vi "Project Save As.vi"(8 "error in (no error)":errorcluster, 9 "Rename Paths[]":T1[](array[typedef]), 10 "Existing Project Path":path, 11 "New Project Path":path) -> (0 "error out":errorcluster)   [LabVIEW 2016, in "SLL Scripting.lvlib"]
uses:
  SLL Scripting.lvlib
  _Typedefs/Rename Item Cluster.ctl
  <vilib>/Utility/EditLVProj/Edit LVProj.lvlib
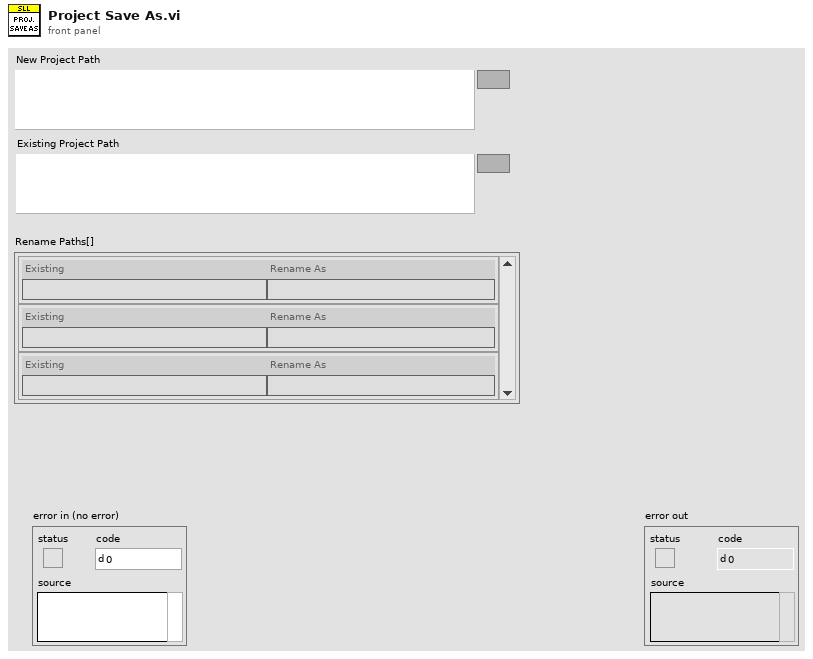
[diagram p1: front panel]
types:
  T1 = typedef "Rename Item Cluster.ctl" = cluster{"Existing":string, "Rename As":string}
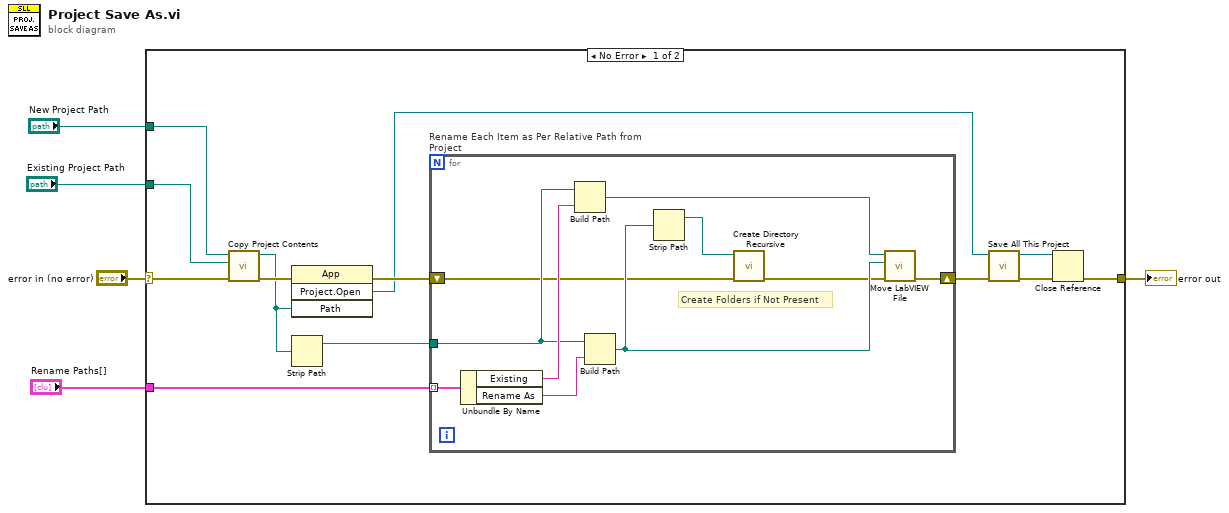
[diagram p0: block diagram]
diagram:
  n1 = case shown="No Error" "error in (no error)" {
    selector: "error in (no error)" -> [w18 w29]
    tunnel: [w7 w29] -> w4
    tunnel: "Existing Project Path" -> [w16 _]
    tunnel: "New Project Path" -> [w17 _]
    tunnel: "Rename Paths[]" -> [w13 _]
    frame No Error {
      n2 = call "Copy Project Contents.vi"("error in (no error)"=w18, "Existing Project Path"=w16, "New Project Path"=w17) -> ("error out"=w15:errorcluster, "New Project Path Out"=w12:path)  [unwired: 7 in]
      n3 = invoke class="App" method="Project.Open"(error in=w15, "Path"=w12) -> (error out=w14:errorcluster, "Project:Open"=w8:refnum<vi>)  [unwired: 2 in, 2 out]
      n4 = Strip Path(path=w12) -> (stripped path=w11:path)  [unwired: 1 out]
      n5 = for "Rename Each Item as Per Relative Path from Project" {
        shift-right: [w23] -> w10
        shift-left: w14 -> [w21]
        tunnel: w13 -> [w28] mode=indexing
        tunnel: w11 -> [w26]
        # "Create Folders if Not Present"
        n6 = Unbundle By Name(w28) -> ("Existing"=w27:string, "Rename As"=w25:string)
        n7 = Build Path(base path=w26, name or relative path=w27) -> (appended path=w24:path)
        n8 = Build Path(base path=w26, name or relative path=w25) -> (appended path=w22:path)
        n9 = Strip Path(path=w22) -> (stripped path=w19:path)  [unwired: 1 out]
        n10 = call <vilib>:"Create Directory Recursive.vi"("error in (no error)"=w21, "directory"=w19) -> ("error out"=w20:errorcluster)  [unwired: 3 in, 2 out]
        n11 = call "Move LabVIEW File.vi"("error in (no error)"=w20, "New Path"=w22, "Existing Path"=w24) -> ("error out"=w23:errorcluster)  [unwired: 8 in]
      }
      n12 = call <vilib>:"Save All This Project.vi"("error in (no error)"=w10, "Project in"=w8) -> ("error out"=w9:errorcluster, "Project out"=w6:refnum<vi>)  [unwired: 8 in]
      n13 = Close Reference(reference=w6, error in (no error)=w9) -> (error out=w7:errorcluster)
    }
    frame Error {
    }
  }
  "error out" <- w4
